vi "Using Meshes.vi"() -> ()   [LabVIEW 2023]
doc: "This example demonstrates how to apply a mesh to an object that appears in a 3D picture control. The values you set for the SceneMesh:Set Mesh Parameters method determine how LabVIEW renders the object to which you apply the mesh."
uses:
  <vilib>/Utility/miscctls.llb/LV3DPointTypeDef.ctl
  <vilib>/picture/3D Picture Control/Object/Create Object (drawable with reference).vi
  <vilib>/picture/3D Picture Control/Object/Create Object (name).vi
  <vilib>/picture/3D Picture Control/Helpers/Apply Texture (no reference).vi
  <vilib>/picture/3D Picture Control/Object/Add Object (no reference).vi
  <vilib>/picture/3D Picture Control/Helpers/Set Light (reference).vi
  <vilib>/picture/3D Picture Control/NI_3D Picture Control.lvlib
panel:
  in  "Texturing":enum16{"Inherit Value", "Off", "On"}(ring)=enum."On"
  out "3D Picture":refnum<vi>(3d-picture)
  in  "Z":dbl(knob)=-1.9091030626789895 scale=-5.0..5.0
  in  "Y":dbl(knob) scale=-5.0..5.0
  in  "X":dbl(knob)=-0.3580264266875792 scale=-5.0..5.0
  in  "Light On?":bool=TRUE
  out "Example of Expected Vertex Order":picture
  in  "Draw Style Mode":u16(ring)=3 items=["Inherit Value", "Points", "Wireframe", "Polygons"]
  in  "Stop":bool
  in  "Normal Binding Mode":u16(ring) items=["Overall", "Per Primitive", "Per Vertex", "Binding Off"]
  in  "Color Binding Mode":u16(ring) items=["Overall", "Per Primitive", "Per Vertex", "Binding Off"]
  in  "Draw Mode":u16(ring)=4 items=["Points", "Lines", "Line Strip", "Line Loop", "Triangles", "Triangle Strip", "Triangle Fan", "Quads", "Quad Strip", "Polygon"]
  # "Overview: Demonstrates how to create your own shape in a 3D Picture by using a polygon mesh.\nRequirements: LabVIEW Full Development System\nInstructions: \n1. Run the VI.\n2. Select different modes from the Draw Mode ring. The Example of Expected Vertex Order image displays the different ways LabVIEW can draw the polygon across the vertices of the 3D object.\n3. Select different modes from the Normal Binding Mode, Color Binding Mode, and Draw Style Mode rings to see how each mode affects the rendering of the 3D object.\n4. Change the Texturing value to see how the appearance of the 3D object changes when you apply texture.\n5. Turn the X, Y, and Z knobs to see how changing the position of a light source affects the appearance of the 3D object.\n6. Click Stop to stop the VI."
  # "Light Position"
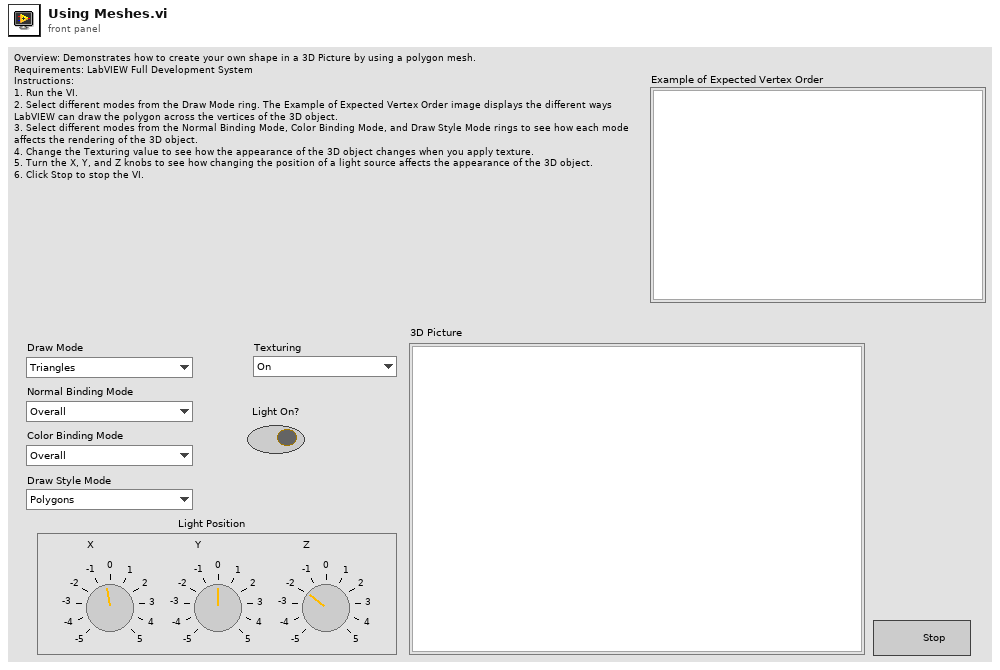
[diagram p1: front panel]
types:
  T1 = typedef "LV3DPointTypeDef.ctl" = cluster{"X":sgl, "Y":sgl, "Z":sgl}
  T2 = cluster{"number: 0 to 1":dbl, "number: 0 to 1":dbl, "number: 0 to 1":dbl, "Alpha":dbl}[]
  T3 = typedef "imagedata.ctl" = cluster{"image type":i32, "image depth":i32, "image":u8[], "mask":u8[], "colors":u32[], "Rectangle":cluster{"left":i16, "top":i16, "right":i16, "bottom":i16}}
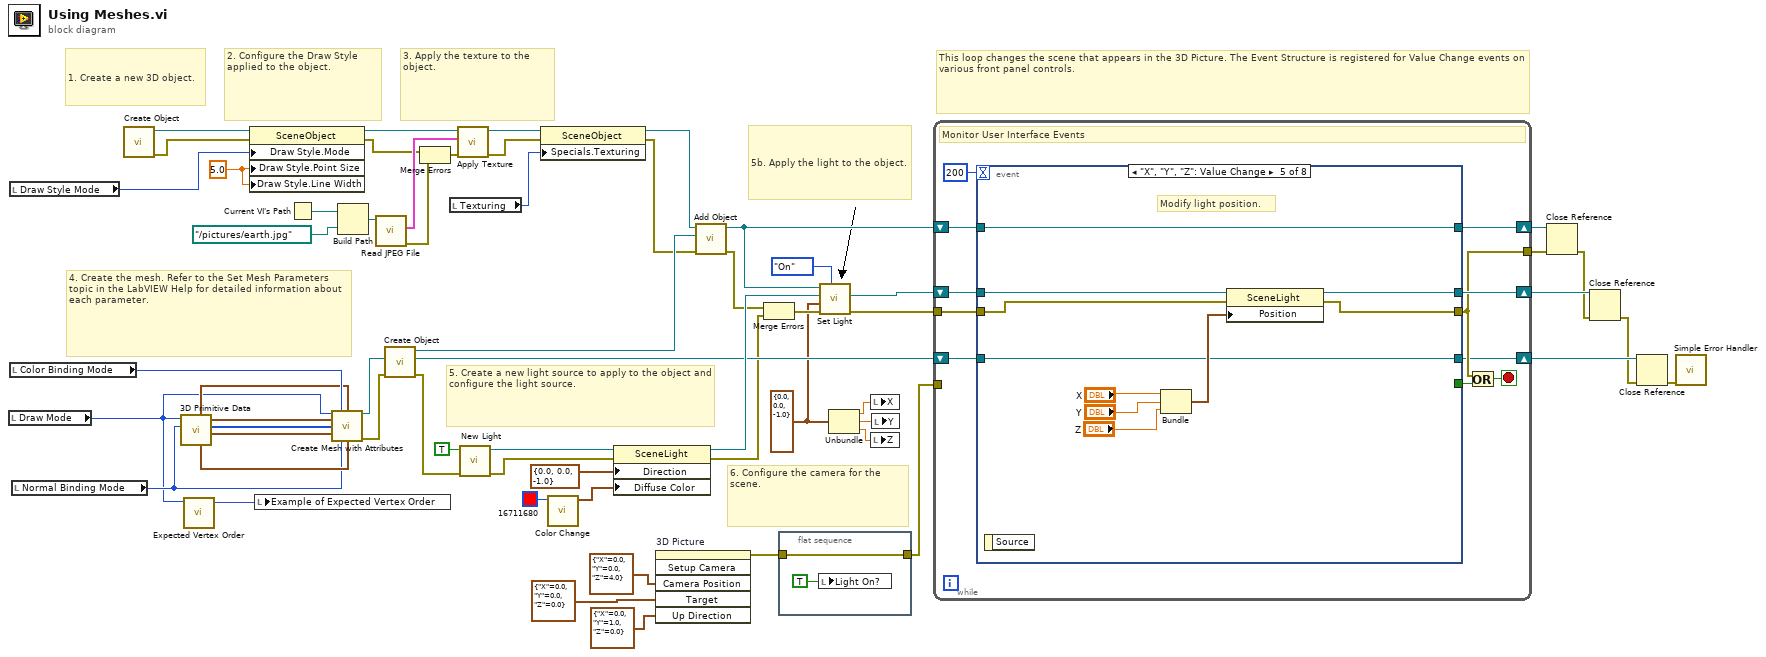
[diagram p0: block diagram]
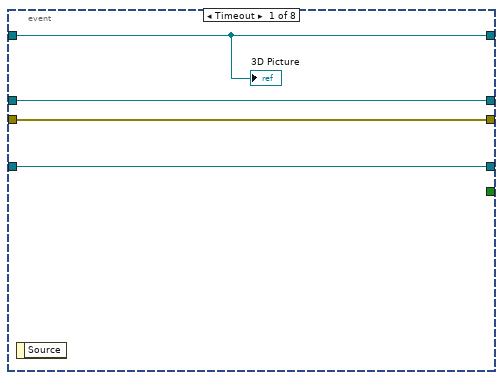
[diagram p2: hidden frame]
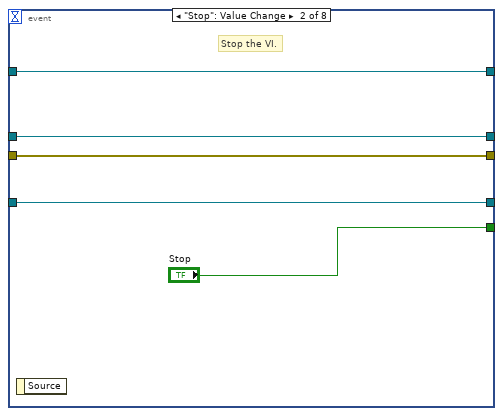
[diagram p3: hidden frame]
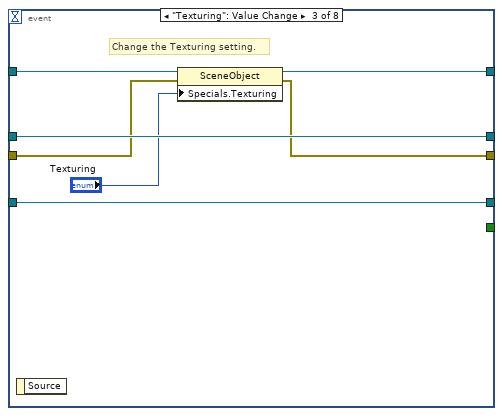
[diagram p4: hidden frame]
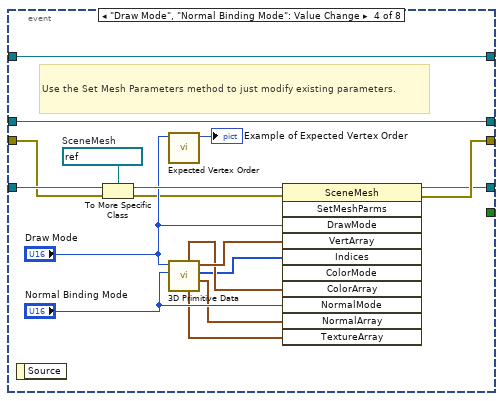
[diagram p5: hidden frame]
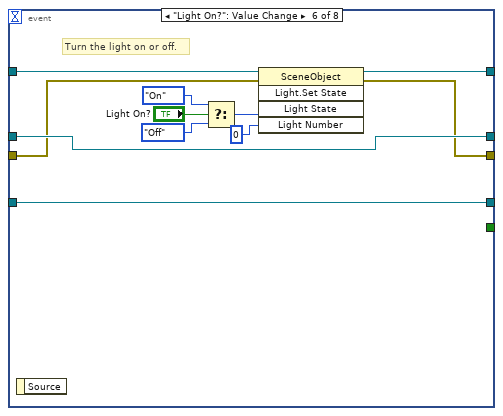
[diagram p6: hidden frame]
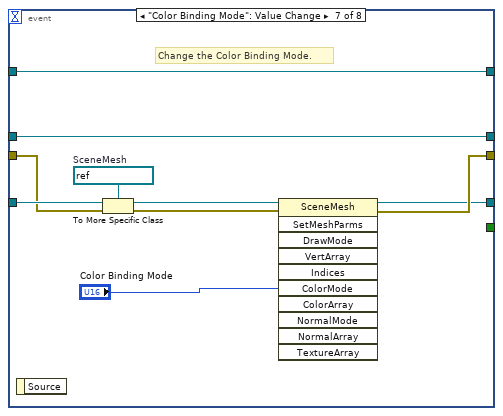
[diagram p7: hidden frame]
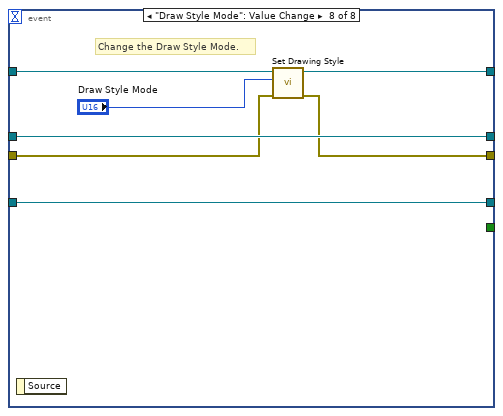
[diagram p8: hidden frame]
diagram:
  w17 = T1 {"X"=0.0, "Y"=0.0, "Z"=-1.0} ("Position")
  w27 = sgl 5.0 ("Draw Style:Point Size")
  # "6. Configure the camera for the scene."
  # "5b. Apply the light to the object."
  # "5. Create a new light source to apply to the object and configure the light source."
  # "4. Create the mesh. Refer to the Set Mesh Parameters topic in the LabVIEW Help for detailed information about each parameter."
  # "3. Apply the texture to the object."
  # "2. Configure the Draw Style applied to the object."
  # "1. Create a new 3D object."
  # "This loop changes the scene that appears in the 3D Picture. The Event Structure is registered for Value Change events on various front panel controls."
  n1 = local read "Draw Mode"() -> (w22:u16)
  n2 = local read "Draw Style Mode"() -> (w28:u16)
  n3 = local read "Color Binding Mode"() -> (w47:u16)
  n4 = local read "Normal Binding Mode"() -> (w45:u16)
  n5 = call-poly <vilib>:"Create Object.vi"() -> ("error out"=w25:errorcluster, "Scene:New Object"=w29:refnum<vi>)  [unwired: 10 in]
  n6 = call "3D Primitive Data.vi"("Normal Binding Mode"=w45, "Primitive Mode"=w22) -> ("Normal Array"=w32:cluster{"X":sgl, "Y":sgl, "Z":sgl}[], "Indices"=w48:u32[], "Vertex Array"=w49:cluster{"X":sgl, "Y":sgl, "Z":sgl}[], "Texture Array"=w46:cluster{"X":sgl, "Y":sgl}[], "Color Array"=w33:T2)  [unwired: 5 out]
  n7 = call "Expected Vertex Order.vi"("Draw Mode"=w22) -> ("Picture"=w56:picture)  [unwired: 10 in]
  n8 = property class="SceneObject"(reference=w29, error in=w25, "Draw Style.Mode"=w28, "Draw Style.Point Size"=w27, "Draw Style.Line Width"=w27) -> (reference out=w26:refnum<vi>, error out=w13:errorcluster)
  n9 = local write "Example of Expected Vertex Order"(w56) -> ()
  n10 = Current VI's Path() -> (path=w9:path)
  n11 = call <vilib>:"Create Mesh with Attributes.vi"("Draw Mode"=w22, "Color Binding Mode"=w47, "Color Array"=w33, "Vertex Array"=w49, "Indices"=w48, "Normal Array"=w32, "Normal Binding Mode"=w45, "Texture Coordinate Array"=w46) -> ("New Mesh Refnum"=w42:refnum<vi>, "error out"=w31:errorcluster)  [unwired: 6 in]
  n12 = Build Path(base path=w9, name or relative path=path "../pictures/earth.jpg" ("stripped path")) -> (appended path=w44:path)
  n13 = call <vilib>:"Read JPEG File.vi"("path to JPEG file"=w44) -> ("error out"=w11:errorcluster, "image data"=w60:T3)  [unwired: 1 in, 8 out]
  n14 = call-poly <vilib>:"Create Object.vi"("error in (no error)"=w31, "Geometry or text"=w42) -> ("error out"=w23:errorcluster, "Drawable refnum"=w39:refnum<vi>, "Scene:New Object"=w41:refnum<vi>)  [unwired: 7 in]
  n15 = Merge Errors(w13, w11) -> (w12:errorcluster)
  n16 = local read "Texturing"() -> (w37:enum16{"Inherit Value", "Off", "On"})
  n17 = call-poly <vilib>:"Apply Texture.vi"("error in (no error)"=w12, "Image Data"=w60, "Scene Object In"=w26) -> ("error out"=w35:errorcluster, "Scene Object Out"=w38:refnum<vi>)  [unwired: 7 in]
  n18 = call <vilib>:"New Light.vi"("error in (no error)"=w23, "At Infinity"=TRUE) -> ("error out"=w24:errorcluster, "New Light Refnum"=w59:refnum<vi>)  [unwired: 1 in, 7 out]
  n19 = property class="SceneObject"(reference=w38, error in=w35, "Specials.Texturing"=w37) -> (reference out=w36:refnum<vi>, error out=w34:errorcluster)
  n20 = call <vilib>:"Color Change.vi"("Color"=u32 16711680) -> ("RGBA"=w10:cluster{"R":sgl, "G":sgl, "B":sgl, "A":sgl})  [unwired: 10 in]
  n21 = property class="SceneLight"(reference=w59, error in=w24, "Direction"=cluster{"X":sgl, "Y":sgl, "Z":sgl} {"X"=0.0, "Y"=0.0, "Z"=-1.0}, "Diffuse Color"=w10) -> (reference out=w50:refnum<vi>, error out=w20:errorcluster)
  n22 = invoke on="3D Picture" class="SceneGraphDisp (strict)" method="Setup Camera"("Camera Position"=cluster{"X":sgl, "Y":sgl, "Z":sgl} {"X"=0.0, "Y"=0.0, "Z"=4.0} ("Up Direction"), "Target"=cluster{"X":sgl, "Y":sgl, "Z":sgl} {"X"=0.0, "Y"=0.0, "Z"=0.0} ("Up Direction"), "Up Direction"=cluster{"X":sgl, "Y":sgl, "Z":sgl} {"X"=0.0, "Y"=1.0, "Z"=0.0}) -> (error out=w53:errorcluster)  [unwired: 3 in, 5 out]
  n23 = call-poly <vilib>:"Add Object.vi"("error in (no error)"=w34, "New Object In"=w41, "Scene Object In"=w36) -> ("error out"=w19:errorcluster, "Scene Object Out"=w40:refnum<vi>)  [unwired: 7 in]
  n24 = Merge Errors(w19, w20) -> (w21:errorcluster)
  n25 = flat-sequence {
    tunnel: w53 -> [w62]
    tunnel: [w62] -> w52
    frame #0 {
      n26 = local write "Light On?"(TRUE ("Light On?")) -> ()
    }
  }
  n27 = call-poly <vilib>:"Set Light.vi"("Light State"=enum16{"Inherit Value", "Off", "On"}."On", "error in (no error)"=w21, "Position"=w17, "Light Refnum In"=w50, "Scene Object In"=w40) -> ("error out"=w18:errorcluster, "Light Refnum Out"=w1:refnum<vi>)  [unwired: 4 in, 1 out]
  n28 = Unbundle(w17) -> ("X"=w16:sgl, "Y"=w15:sgl, "Z"=w14:sgl)
  n29 = local write "X"(w16) -> ()
  n30 = local write "Z"(w14) -> ()
  n31 = local write "Y"(w15) -> ()
  n32 = while {
    tunnel: w52 -> [_]
    shift-right: [w69] -> w8
    shift-left: w1 -> [w70]
    tunnel: w18 -> [w68]
    tunnel: [w66] -> w5
    shift-right: [w65] -> w7
    shift-left: w39 -> [w71]
    shift-right: [w64] -> w6
    shift-left: w40 -> [w74]
    stop <- w67 stop-if-true
    # "Monitor User Interface Events"
    n33 = event shown="[4] \"X\", \"Y\", \"Z\": Value Change" {
      selector: _ -> [_ _ _ _ _ _ _ _]
      dyn-events: _ -> [_ _ _ _ _ _ _ _]
      timeout: 200 -> [_ _ _ _ _ _ _ _]
      tunnel: w74 -> [w75 w79 w90 w91 w108 w128 w129 w144]
      tunnel: [_ "Stop" _ _ _ _ _ _] -> w72
      tunnel: w71 -> [w76 w80 w85 w107 w109 w119 w138 w140]
      tunnel: w70 -> [w78 w82 w89 w103 w117 w127 w135 w145]
      tunnel: [w78 w82 w89 w103 w112 w127 w135 w145] -> w69
      tunnel: w68 -> [w77 w81 w87 w96 w111 w121 w133 w142]
      tunnel: [w77 w81 w86 w94 w110 w120 w131 w141] -> w66
      tunnel: [w76 w80 w85 w92 w109 w119 w130 w140] -> w65
      tunnel: [w75 w79 w84 w91 w108 w118 w129 w139] -> w64
      event Timeout {
        n34 = event-data() -> ()  [unwired: 2 out]
        "3D Picture" <- w75
      }
      event "Stop": Value Change {
        # "Stop the VI."
        n35 = event-data() -> ()  [unwired: 2 out]
      }
      event "Texturing": Value Change {
        # "Change the Texturing setting."
        n36 = event-data() -> ()  [unwired: 2 out]
        n37 = property class="SceneObject"(reference=w90, error in=w87, "Specials.Texturing"="Texturing") -> (reference out=w84:refnum<vi>, error out=w86:errorcluster)
      }
      event "Draw Mode", "Normal Binding Mode": Value Change {
        w106 = refnum<vi> refnum  # SceneMesh
        # "Use the Set Mesh Parameters method to just modify existing parameters."
        n38 = event-data() -> ()  [unwired: 2 out]
        n39 = To More Specific Class(target class=w106, reference=w107, error in=w96) -> (specific class reference=w105:refnum<vi>, error out=w95:errorcluster)
        n40 = call "Expected Vertex Order.vi"("Draw Mode"="Draw Mode") -> ("Picture"=→"Example of Expected Vertex Order":picture)  [unwired: 10 in]
        n41 = call "3D Primitive Data.vi"("Normal Binding Mode"="Normal Binding Mode", "Primitive Mode"="Draw Mode") -> ("Normal Array"=w97:cluster{"X":sgl, "Y":sgl, "Z":sgl}[], "Indices"=w93:u32[], "Vertex Array"=w100:cluster{"X":sgl, "Y":sgl, "Z":sgl}[], "Texture Array"=w99:cluster{"X":sgl, "Y":sgl}[], "Color Array"=w98:T2)  [unwired: 5 out]
        n42 = invoke class="SceneMesh" method="SetMeshParms"(reference=w105, error in=w95, "DrawMode"="Draw Mode", "VertArray"=w100, "Indices"=w93, "ColorArray"=w98, "NormalMode"="Normal Binding Mode", "NormalArray"=w97, "TextureArray"=w99) -> (reference out=w92:refnum<vi>, error out=w94:errorcluster)  [unwired: 2 in, 9 out]
      }
      event "X", "Y", "Z": Value Change {
        # "Modify light position."
        n43 = event-data() -> ()  [unwired: 2 out]
        n44 = Bundle("X"="X", "Y"="Y", "Z"="Z") -> (w113:cluster{"X":dbl, "Y":dbl, "Z":dbl})  [unwired: 1 out]
        n45 = property class="SceneLight"(reference=w117, error in=w111, "Position"=w113) -> (reference out=w112:refnum<vi>, error out=w110:errorcluster)
      }
      event "Light On?": Value Change {
        # "Turn the light on or off."
        n46 = event-data() -> ()  [unwired: 2 out]
        n47 = Select(t=enum16{"Inherit Value", "Off", "On"}."On" ("Light State"), s="Light On?", f=enum16{"Inherit Value", "Off", "On"}."Off" ("Light State")) -> (s? t:f=w122:enum16{"Inherit Value", "Off", "On"})
        n48 = invoke class="SceneObject" method="Light.Set State"(reference=w128, error in=w121, "Light State"=w122, "Light Number"=0) -> (reference out=w118:refnum<vi>, error out=w120:errorcluster)  [unwired: 1 in, 3 out]
      }
      event "Color Binding Mode": Value Change {
        w137 = refnum<vi> refnum  # SceneMesh
        # "Change the Color Binding Mode."
        n49 = event-data() -> ()  [unwired: 2 out]
        n50 = To More Specific Class(target class=w137, reference=w138, error in=w133) -> (specific class reference=w136:refnum<vi>, error out=w132:errorcluster)
        n51 = invoke class="SceneMesh" method="SetMeshParms"(reference=w136, error in=w132, "ColorMode"="Color Binding Mode") -> (reference out=w130:refnum<vi>, error out=w131:errorcluster)  [unwired: 8 in, 9 out]
      }
      event "Draw Style Mode": Value Change {
        # "Change the Draw Style Mode."
        n52 = event-data() -> ()  [unwired: 2 out]
        n53 = call <vilib>:"Set Drawing Style.vi"("error in (no error)"=w142, "Mode"="Draw Style Mode", "Scene Object In"=w144) -> ("error out"=w141:errorcluster, "Scene Object Out"=w139:refnum<vi>)  [unwired: 7 in]
      }
    }
    n54 = Or(x=w66, y=w72) -> (x .or. y?=w67:bool)
  }
  n55 = Close Reference(reference=w6, error in (no error)=w5) -> (error out=w4:errorcluster)
  n56 = Close Reference(reference=w8, error in (no error)=w4) -> (error out=w3:errorcluster)
  n57 = Close Reference(reference=w7, error in (no error)=w3) -> (error out=w2:errorcluster)
  n58 = call <vilib>:"Simple Error Handler.vi"("error in (no error)"=w2) -> ()  [unwired: 4 in, 5 out]
